vi "populate listbox with available tags.vi"(7 "instance id":string, 8 "error in":errorcluster, 9 "channel":refnum<class "TBM channel.lvclass">, 10 "CtlRef":refnum<vi>, 11 "engine configuration in":refnum<class "engine configuration.lvclass">) -> (0 "error out":errorcluster, 3 "engine configuration out":refnum<class "engine configuration.lvclass">)   [LabVIEW 2013, in "tag bus processing plugin editor node.lvclass"]
uses:
  tag bus processing plugin editor node.lvclass
  <vilib>/NI/Tag Bus Module Framework/channel/TBM channel.lvclass
  <vilib>/NI/Module Execution Interface/Engine Configuration/engine configuration.lvclass
  <vilib>/NI/Tag Bus Module Framework/channel/TBM channel.lvclass/TBM channel.ctl
  <vilib>/NI/Tag Bus/tag/tag descriptor.lvclass
  <vilib>/NI/Tag Bus/tag/tag descriptor.lvclass/tag descriptor.ctl
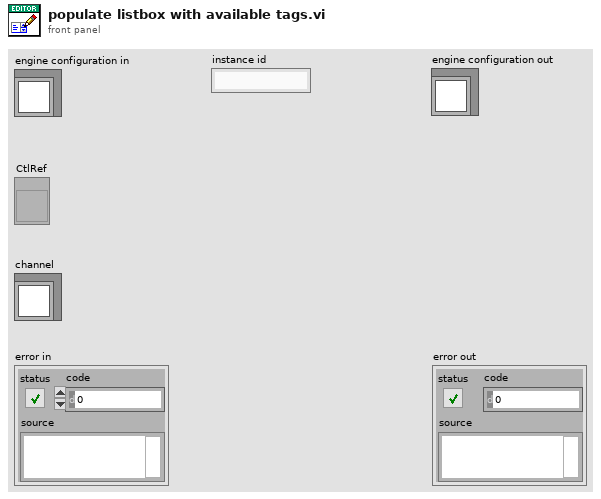
[diagram p1: front panel]
types:
  T1 = typedef "TBM channel.lvclass/channel classification.ctl" = enum16{"input data", "output data", "processing parameter", "processing result"}
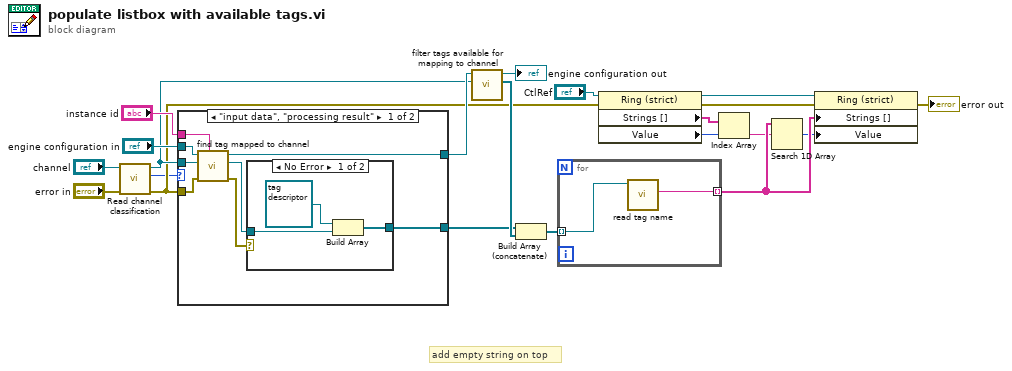
[diagram p0: block diagram]
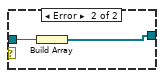
[diagram p2: hidden frame]
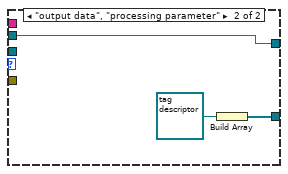
[diagram p3: hidden frame]
diagram:
  # "add empty string on top"
  n1 = call <vilib>:"Read channel classification.vi"("error in"="error in", "channel in"="channel") -> ("error out"=w10:errorcluster, "channel classification"=w9:T1, "channel out"=w12:refnum<class "TBM channel.lvclass">)  [unwired: 7 in]
  n2 = case shown="\"input data\", \"processing result\"" w9 {
    tunnel: "instance id" -> [w29 _]
    tunnel: [w28 w35] -> w20
    tunnel: "engine configuration in" -> [w27 w35]
    tunnel: [w24 w36] -> w14
    tunnel: w12 -> [w23 _]
    tunnel: w10 -> [w22 _]
    frame "input data", "processing result" {
      n3 = call <vilib>:"find tag mapped to channel.vi"("owner"=w29, "error in"=w22, "channel"=w23, "engine configuration in"=w27) -> ("error out"=w26:errorcluster, "tag"=w25:refnum<class "tag descriptor.lvclass">, "engine configuration out"=w28:refnum<class "engine configuration.lvclass">)  [unwired: 5 in]
      n4 = case shown="No Error" w26 {
        tunnel: w25 -> [w32 w33]
        tunnel: [w30 w34] -> w24
        frame No Error {
          n5 = Build Array(refnum<class "tag descriptor.lvclass"> refnum ("tag"), w32) -> (w30:refnum<class "tag descriptor.lvclass">[])
        }
        frame Error {
          n6 = Build Array(w33) -> (w34:refnum<class "tag descriptor.lvclass">[])
        }
      }
    }
    frame "output data", "processing parameter" {
      n7 = Build Array(refnum<class "tag descriptor.lvclass"> refnum ("tag")) -> (w36:refnum<class "tag descriptor.lvclass">[])
    }
  }
  n8 = call <vilib>:"filter tags available for mapping to channel.vi"("channel to map to"=w12, "engine configuration in"=w20) -> ("filtered tags"=w16:refnum<class "tag descriptor.lvclass">[], "engine configuration out"=→"engine configuration out":refnum<class "engine configuration.lvclass">)  [unwired: 8 in]
  n9 = Build Array (concatenate)(w14, w16) -> (w17:refnum<class "tag descriptor.lvclass">[])
  n10 = for {
    tunnel: w17 -> [w38] mode=indexing
    tunnel: [w39] -> w3 mode=indexing
    n11 = call <vilib>:"read tag name.vi"("system tag in"=w38) -> ("name"=w39:string)  [unwired: 8 in, 2 out]
  }
  n12 = property class="Ring (strict)"(reference="CtlRef", error in=w10) -> (reference out=w4:refnum<vi>, error out=w8:errorcluster, "Strings []"=w6:string[], "Value"=w5:u16)
  n13 = Index Array(array=w6, index=w5) -> (element=w2:string)
  n14 = Search 1D Array(1D array=w3, element=w2) -> (index of element=w1:i32)  [unwired: 1 in]
  n15 = property on="Property Node" class="Ring (strict)"(reference=w4, error in=w8, "Strings []"=w3, "Value"=w1) -> (error out=→"error out":errorcluster)  [unwired: 1 out]
